vi "BCM_Light_Str.vi"(1 "BCM_Light":T1 {"BCM指示转向拔杆状态" items=["Inactive", "Turn left", "Turn right", "Error status"]}) -> (0 "CmdStr":string)   [LabVIEW 2013]
uses:
  BCM_Ligh_1F0.ctl
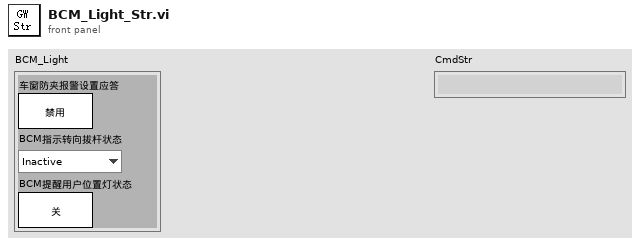
[diagram p1: front panel]
types:
  T1 = typedef "BCM_Ligh_1F0.ctl" = cluster{"车窗防夹报警设置应答":bool, "BCM指示转向拔杆状态":u16, "BCM提醒用户位置灯状态":bool}
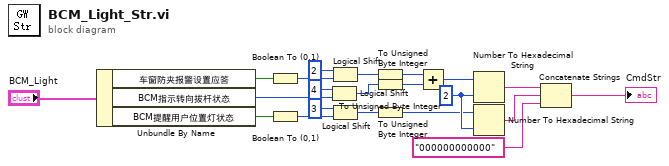
[diagram p0: block diagram]
diagram:
  w4 = i16 2 ("y")
  n1 = Unbundle By Name("BCM_Light") -> ("车窗防夹报警设置应答"=w19:bool, "BCM指示转向拔杆状态"=w15:u16, "BCM提醒用户位置灯状态"=w8:bool)
  n2 = Boolean To (0,1)(Boolean=w19) -> (0, 1=w18:i16)
  n3 = Boolean To (0,1)(Boolean=w8) -> (0, 1=w7:i16)
  n4 = Logical Shift(y=i16 4, x=w15) -> (x << y=w13:u16)
  n5 = Logical Shift(y=i16 2, x=w18) -> (x << y=w16:i16)
  n6 = Logical Shift(y=i16 3, x=w7) -> (x << y=w5:i16)
  n7 = To Unsigned Byte Integer(number=w16) -> (unsigned 8bit integer=w12:u8)
  n8 = To Unsigned Byte Integer(number=w13) -> (unsigned 8bit integer=w6:u8)
  n9 = To Unsigned Byte Integer(number=w5) -> (unsigned 8bit integer=w3:u8)
  n10 = Add(x=w12, y=w6) -> (x+y=w11:u8)
  n11 = Number To Hexadecimal String(1:w4, 2:w11) -> (0:w10:string)
  n12 = Number To Hexadecimal String(1:w4, 2:w3) -> (0:w2:string)
  n13 = Concatenate Strings(w10, w2, "000000000000") -> (→"CmdStr":string)
